vi "8-bit video export-setup.vi"(7 "Funct data?":bool) -> (1 "output cluster":T2, 3 "cancelled":bool, 11 "Path":path)   [LabVIEW 2020]
uses:
  <vilib>/vision/Avi.llb/IMAQ AVI2 Refnum.ctl
  Globals/gl_Time series viewer globals.vi
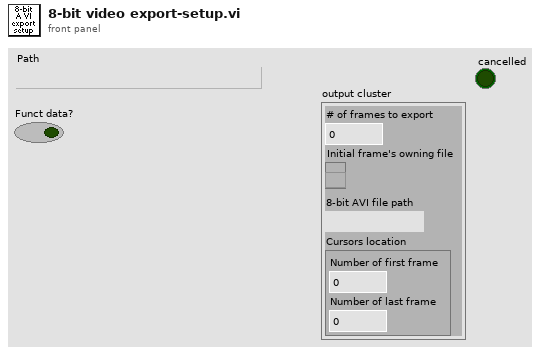
[diagram p1: front panel]
types:
  T1 = typedef "IMAQ AVI2 Refnum.ctl" = refnum<k20>
  T2 = cluster{"# of frames to export":i32, "Initial frame's owning file":T1, "8-bit AVI file path":path, "Cursors location":cluster{"Number of first frame":i32, "Number of last frame":i32}}
  T3 = typedef "Time series viewer refs.ctl" = cluster{"This VI":refnum<vi>, "Image control":refnum<vi>, "AVI Mode ind":refnum<vi>, "Play":refnum<vi>, "Stop":refnum<vi>, "Back":refnum<vi>, "Scrollbar":refnum<vi>, "Video length info":refnum<vi>, "Expected speed values":refnum<vi>, "Intensity":refnum<vi>, "Path":refnum<vi>, "Selection sliders":refnum<vi>, "Speed Graph ref":refnum<vi>, "Frame rate set (fps)":refnum<vi>, "Number of rows to generate":refnum<vi>, "VL Image Array":refnum<vi>, "Image Scrollbar":refnum<vi>, "Channel to load":refnum<vi>, "Colour":refnum<vi>}
  T4 = enum16{"Export from full dataset", "Export from cursors selection"}
  T5 = cluster{"Number of first frame":i32, "Number of last frame":i32}
  T6 = cluster{"Caption-Right button":string, "Caption-Left button":string, "Message to display":string, "Delay before close":u32, "Window Colour":u32, "Cancel button disabled?":enum8{"Enabled", "Disabled", "Disabled and Grayed Out"}}
  T7 = typedef "AVI modes refs cluster.ctl" = cluster{"AVI1 ref":T8, "AVI2 refs":T1[], "AVI # frames":u32[]}
  T8 = typedef "AviRefnum.ctl" = refnum<k1>
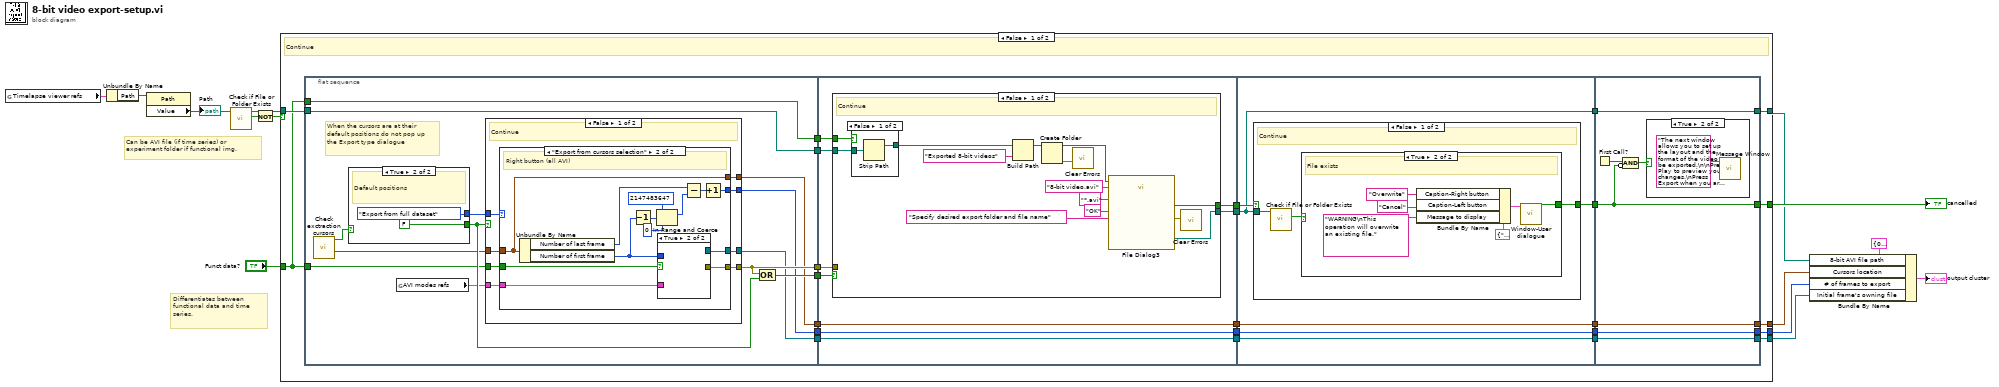
[diagram p0: block diagram]
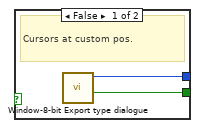
[diagram p2: hidden frame]
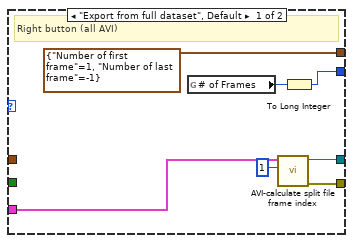
[diagram p3: hidden frame]
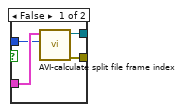
[diagram p4: hidden frame]
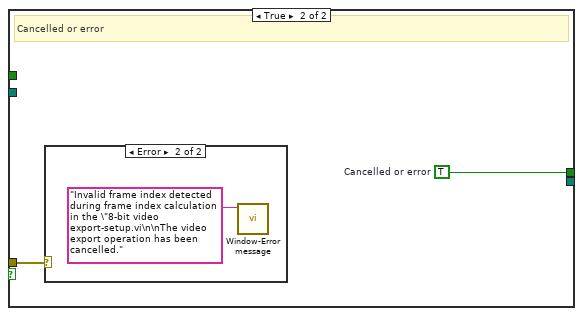
[diagram p7: hidden frame]
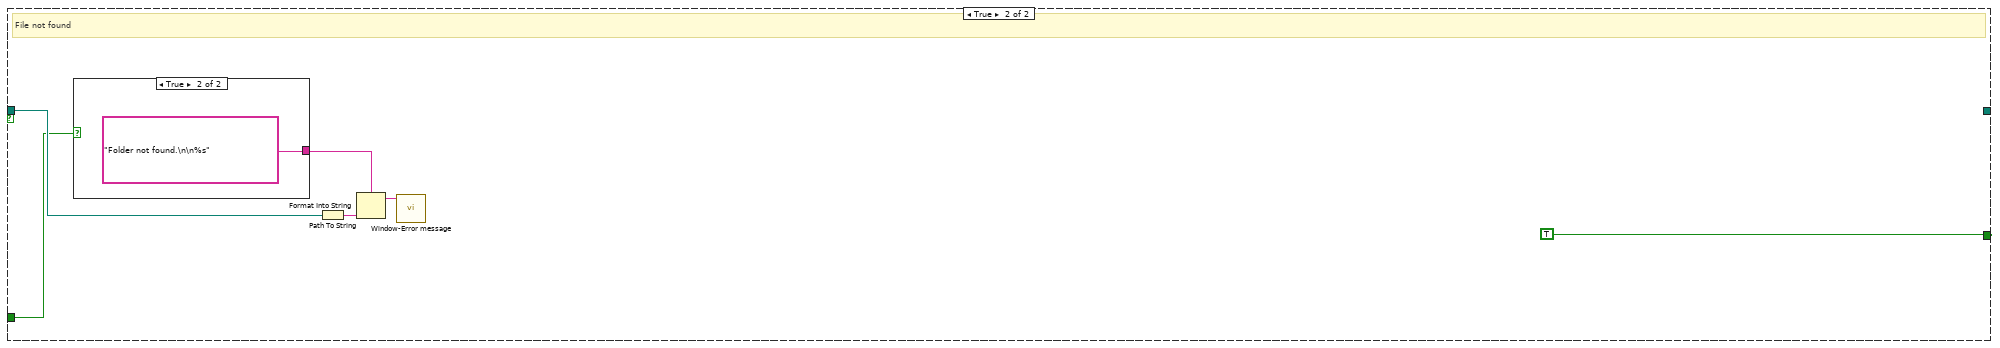
[diagram p12: hidden frame]
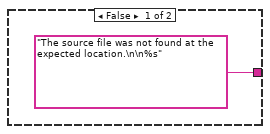
[diagram p13: hidden frame]
diagram:
  # "Differentiates between functional data and time series."
  # "Can be AVI file (if time series) or experiment folder if functional img."
  n1 = global read "gl_Time series viewer globals.vi" "Timelapse viewer refs"() -> (w4:T3)
  n2 = Unbundle By Name(w4) -> ("Path"=w3:refnum<vi>)
  n3 = property class="Path"(reference=w3) -> ("Value"=w2:path)  [unwired: 1 in, 2 out]
  "Path" <- w2
  n4 = call <vilib>:"Check if File or Folder Exists.vi"("path"=w2) -> ("file or folder exists?"=w5:bool, "dup path"=w14:path)  [unwired: 8 in, 1 out]
  n5 = Not(x=w5) -> (.not. x?=w13:bool)
  n6 = case shown="False" w13 {
    tunnel: [w36 _] -> w9
    tunnel: [w35 TRUE ("cancelled")] -> w10
    tunnel: w14 -> [w34 w142]
    tunnel: [w24 _] -> w8
    tunnel: [w23 _] -> w7
    tunnel: [w22 _] -> w6
    tunnel: "Funct data?" -> [w15 w141]
    frame False {
      # "Continue"
      n7 = flat-sequence {
        tunnel: [w50] -> w38
        tunnel: w34 -> [w50]
        tunnel: [w48] -> w32
        tunnel: [w47] -> w31
        tunnel: [w46] -> w29
        tunnel: [w45] -> w28
        tunnel: [w44] -> w26
        tunnel: [w40] -> w16
        tunnel: w15 -> [w40]
        tunnel: w15 -> [w39]
        tunnel: w38 -> [w96]
        tunnel: [w95] -> w37
        tunnel: [w94] -> w33
        tunnel: w32 -> [w93]
        tunnel: w31 -> [w92]
        tunnel: [w91] -> w30
        tunnel: w29 -> [w91]
        tunnel: w28 -> [w90]
        tunnel: [w90] -> w27
        tunnel: w26 -> [w89]
        tunnel: [w89] -> w25
        tunnel: w16 -> [w88]
        tunnel: w37 -> [w122]
        tunnel: w33 -> [w117]
        tunnel: w30 -> [w119]
        tunnel: w27 -> [w118]
        tunnel: w25 -> [w120]
        tunnel: [w117] -> w21
        tunnel: [w121] -> w20
        tunnel: [w120] -> w19
        tunnel: [w119] -> w18
        tunnel: [w118] -> w17
        tunnel: [w136] -> w22
        tunnel: [w137] -> w23
        tunnel: [w138] -> w24
        tunnel: [w134] -> w35
        tunnel: [w139] -> w36
        tunnel: w21 -> [w139]
        tunnel: w20 -> [w134]
        tunnel: w19 -> [w138]
        tunnel: w18 -> [w137]
        tunnel: w17 -> [w136]
        frame #0 {
          # "When the cursors are at their default positions do not pop up the Export type dialogue"
          n8 = call "Check exctraction cursors.vi"() -> ("Cursors positions"=w43:T5, "Extraction cursors at default positions"=w42:bool)  [unwired: 9 in, 1 out]
          n9 = case shown="True" w42 {
            tunnel: [w53 T4."Export from full dataset" ("Export type")] -> w51
            tunnel: [w52 FALSE ("Cancelled")] -> w49
            frame False {
              # "Cursors at custom pos."
              n10 = call "Window-8-bit Export type dialogue.vi"() -> ("Cancelled"=w52:bool, "Export type"=w53:T4)  [unwired: 10 in]
            }
            frame True {
              # "Default positions"
            }
          }
          n11 = global read "gl_Time series viewer globals.vi" "AVI modes refs"() -> (w41:T7)
          n12 = case shown="False" w49 {
            tunnel: w51 -> [w63 _]
            tunnel: [w62 _] -> w44
            tunnel: [w58 _] -> w46
            tunnel: w41 -> [w61 _]
            tunnel: [w60 _] -> w47
            tunnel: [w59 _] -> w45
            tunnel: w43 -> [w57 _]
            tunnel: w39 -> [w56 _]
            frame False {
              # "Continue"
              n13 = case shown="\"Export from cursors selection\"" w63 {
                tunnel: [w65 w71] -> w58
                tunnel: [w69 w82] -> w62
                tunnel: w61 -> [w64 w83]
                tunnel: [w67 w76] -> w60
                tunnel: [T5 {"Number of first frame"=1, "Number of last frame"=-1} ("Cursors location") w73] -> w59
                tunnel: w57 -> [_ w73]
                tunnel: w56 -> [_ w72]
                frame "Export from full dataset", Default {
                  # "Right button (all AVI)"
                  n14 = global read "gl_Time series viewer globals.vi" "# of Frames"() -> (w70:u32)
                  n15 = call "AVI-calculate split file frame index.vi"("Frame number (unity-based) in"=1, "AVI modes refs"=w64) -> ("error out"=w67:errorcluster, "AVI2 split file ref"=w69:T1)  [unwired: 6 in, 2 out]
                  n16 = To Long Integer(number=w70) -> (32bit integer=w65:i32)
                }
                frame "Export from cursors selection" {
                  # "Right button (all AVI)"
                  n17 = Unbundle By Name(w73) -> ("Number of last frame"=w75:i32, "Number of first frame"=w74:i32)
                  n18 = Decrement(x=w74) -> (x-1=w80:i32)
                  n19 = In Range and Coerce(upper limit=2147483647, x=w80, lower limit=0) -> (coerced(x)=w77:i32)  [unwired: 1 out]
                  n20 = case shown="True" w72 {
                    tunnel: w83 -> [w87 _]
                    tunnel: [w86 _] -> w82
                    tunnel: [w85 _] -> w76
                    tunnel: w74 -> [w84 _]
                    frame False {
                      n21 = call "AVI-calculate split file frame index.vi"("Frame number (unity-based) in"=w84, "AVI modes refs"=w87) -> ("error out"=w85:errorcluster, "AVI2 split file ref"=w86:T1)  [unwired: 6 in, 2 out]
                    }
                    frame True {
                    }
                  }
                  n22 = Subtract(x=w75, y=w77) -> (x-y=w81:i32)
                  n23 = Increment(x=w81) -> (x+1=w71:i32)
                }
              }
            }
            frame True {
              # "Cancelled"
            }
          }
          n24 = Compound Arithmetic op=OR(w47, w49) -> (w48:bool)
        }
        frame #1 {
          n25 = case shown="False" w93 {
            tunnel: w96 -> [w110 _]
            tunnel: [w109 w115] -> w95
            tunnel: [w108 _] -> w94
            tunnel: w92 -> [_ w114]
            tunnel: w88 -> [w97 _]
            frame False {
              # "Continue"
              n26 = case shown="False" w97 {
                tunnel: w110 -> [w112 w113]
                tunnel: [w111 w113] -> w102
                frame False {
                  n27 = Strip Path(path=w112) -> (stripped path=w111:path)  [unwired: 1 out]
                }
                frame True {
                }
              }
              n28 = Build Path(base path=w102, name or relative path="Exported 8-bit videos") -> (appended path=w100:path)
              n29 = Create Folder(path (use dialog)=w100) -> (created path=w99:path, error out=w98:errorcluster)  [unwired: 2 in, 1 out]
              n30 = call <vilib>:"Clear Errors.vi"("error in (no error)"=w98) -> ()  [unwired: 5 in, 2 out]
              n31 = call "File Dialog3"("start path"=w99, "prompt"="Specify desired export folder and file name" ("default name"), "button label"="OK", "default name"="8-bit video.avi", "pattern (all files)"="*.avi" ("pattern label")) -> ("selected path"=w108:path, "cancelled"=w109:bool, "error out"=w107:errorcluster)  [unwired: 7 in, 1 out]
              n32 = call <vilib>:"Clear Errors.vi"("error in (no error)"=w107) -> ()  [unwired: 5 in, 2 out]
            }
            frame True {
              w115 = TRUE  # Cancelled or error
              # "Cancelled or error"
              n33 = case shown="Error" w114 {
                frame No Error {
                }
                frame Error {
                  n34 = call "Window-Error message.vi"("Message"="Invalid frame index detected during frame index calculation in the \"8-bit video export-setup.vi\n\nThe video export operation has been cancelled.") -> ()  [unwired: 10 in, 1 out]
                }
              }
            }
          }
        }
        frame #2 {
          n35 = case shown="False" w122 {
            selector: w122 -> [_ w132]
            tunnel: w117 -> [w125 _]
            tunnel: [w123 w132] -> w121
            frame False {
              # "Continue"
              n36 = call <vilib>:"Check if File or Folder Exists.vi"("path"=w125) -> ("file or folder exists?"=w124:bool)  [unwired: 8 in, 2 out]
              n37 = case shown="True" w124 {
                tunnel: [_ w131] -> w123
                frame False {
                  # "File does not exist"
                }
                frame True {
                  # "File exists"
                  n38 = Bundle By Name(cluster=T6 {"Caption-Right button"="", "Caption-Left button"="", "Message to display"="", "Delay before close"=0, "Window Colour"=16448250, "Cancel button disabled?"=enum."Enabled"} ("Input cluster"), "Caption-Right button"="Overwrite" ("T button name (\"OK\")"), "Caption-Left button"="Cancel" ("F button name (\"Cancel\")"), "Message to display"="WARNING\nThis operation will overwrite an existing file." ("Message string")) -> (w128:T6)
                  n39 = call "Window-User dialogue.vi"("Input cluster"=w128) -> ("Left Button (Cancel)"=w131:bool)  [unwired: 10 in]
                }
              }
            }
            frame True {
              # "Cancelled"
            }
          }
        }
        frame #3 {
          n40 = First Call?() -> (First Call?: T/F=w135:bool)
          n41 = Compound Arithmetic op=AND(w135, invert w134) -> (w133:bool)
          n42 = case shown="True" w133 {
            frame False {
            }
            frame True {
              n43 = call "Message Window.vi"("Message string"="The next window allows you to set up the layout and the format of the video to be exported.\n\nPress Play to preview your changes.\nPress Export when you are done." ("Message to display")) -> ()  [unwired: 10 in, 1 out]
            }
          }
        }
      }
    }
    frame True {
      # "File not found"
      n44 = case shown="True" w141 {
        tunnel: ["The source file was not found at the expected location.\n\n%s" ("format string") "Folder not found.\n\n%s" ("format string")] -> w145
        frame False {
        }
        frame True {
        }
      }
      n45 = Path To String(path=w142) -> (string=w144:string)
      n46 = Format Into String(format string=w145, w144) -> (resulting string=w143:string)  [unwired: 2 in, 1 out]
      n47 = call "Window-Error message.vi"("Message"=w143) -> ()  [unwired: 10 in, 1 out]
    }
  }
  "cancelled" <- w10
  n48 = Bundle By Name(cluster=T2 {"# of frames to export"=0, "Initial frame's owning file"=refnum, "8-bit AVI file path"=path "", "Cursors location"={"Number of first frame"=0, "Number of last frame"=0}} ("output cluster"), "8-bit AVI file path"=w9, "Cursors location"=w6, "# of frames to export"=w7, "Initial frame's owning file"=w8) -> (→"output cluster":T2)
